vi "AutoDrive.vi"(7 "Drive Params":T1, 8 "Drive PID":T2={"X Dist"={"PID gains"={"proportional gain (Kc)"=1.0, "integral time (Ti, min)"=0.0, "derivative time (Td, min)"=0.0}, "output range"={"output high"=1.0, "output low"=-1.0}}, "Y Dist"={"PID gains"={"proportional gain (Kc)"=1.0, "integral time (Ti, min)"=0.0, "derivative time (Td, min)"=0.0}, "output range"={"output high"=1.0, "output low"=-1.0}}} {"Y Dist"."output range"."output low" format="%.2f"; "Y Dist"."output range"."output high" format="%.2f"; "Y Dist"."PID gains"."derivative time (Td, min)" format="%.3f"; "Y Dist"."PID gains"."integral time (Ti, min)" format="%.3f"; "Y Dist"."PID gains"."proportional gain (Kc)" format="%.3f"; "X Dist"."output range"."output low" format="%.2f"; "X Dist"."output range"."output high" format="%.2f"; "X Dist"."PID gains"."derivative time (Td, min)" format="%.3f"; "X Dist"."PID gains"."integral time (Ti, min)" format="%.3f"; "X Dist"."PID gains"."proportional gain (Kc)" format="%.3f"}, 11 "Array":dbl[](array[numeric]) format="%0.3f") -> (4 "isFinished":bool)   [LabVIEW 2013]
uses:
  AutoDriveParams.ctl
  Drivetrain/DT Mode.ctl
  Drivetrain/Drivetrain Control.ctl
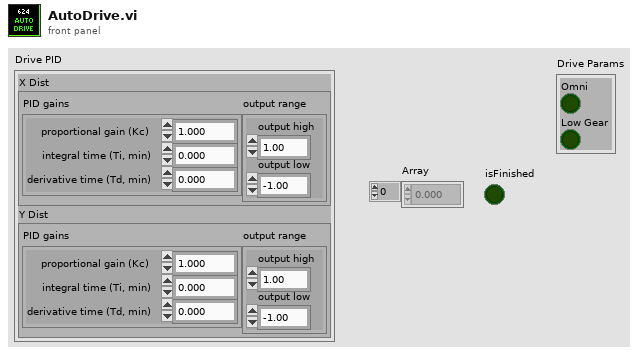
[diagram p1: front panel]
types:
  T1 = typedef "AutoDriveParams.ctl" = cluster{"Omni":bool, "Low Gear":bool}
  T2 = cluster{"X Dist":cluster{"PID gains":cluster{"proportional gain (Kc)":dbl, "integral time (Ti, min)":dbl, "derivative time (Td, min)":dbl}, "output range":cluster{"output high":dbl, "output low":dbl}}, "Y Dist":cluster{"PID gains":cluster{"proportional gain (Kc)":dbl, "integral time (Ti, min)":dbl, "derivative time (Td, min)":dbl}, "output range":cluster{"output high":dbl, "output low":dbl}}}
  T3 = typedef "Drivetrain Control.ctl" = cluster{"axis 1 (x)":dbl, "axis 2 (y)":dbl, "Mode":T4, "heading target":dbl, "steer axis":dbl, "omni?":bool, "Low Gear?":bool, "distance target":cluster{"x":dbl, "y":dbl}, "PID Params":cluster{"X Dist":cluster{"PID gains":cluster{"proportional gain (Kc)":dbl, "integral time (Ti, min)":dbl, "derivative time (Td, min)":dbl}, "output range":cluster{"output high":dbl, "output low":dbl}}, "Y Dist":cluster{"PID gains":cluster{"proportional gain (Kc)":dbl, "integral time (Ti, min)":dbl, "derivative time (Td, min)":dbl}, "output range":cluster{"output high":dbl, "output low":dbl}}}, "Coast":bool}
  T4 = typedef "DT Mode.ctl" = enum16{"Manual", "Gyro Steer", "Distance Drive", "Fieldcentric", "Roll Maneuver", "Alt Roll Maneuver"}
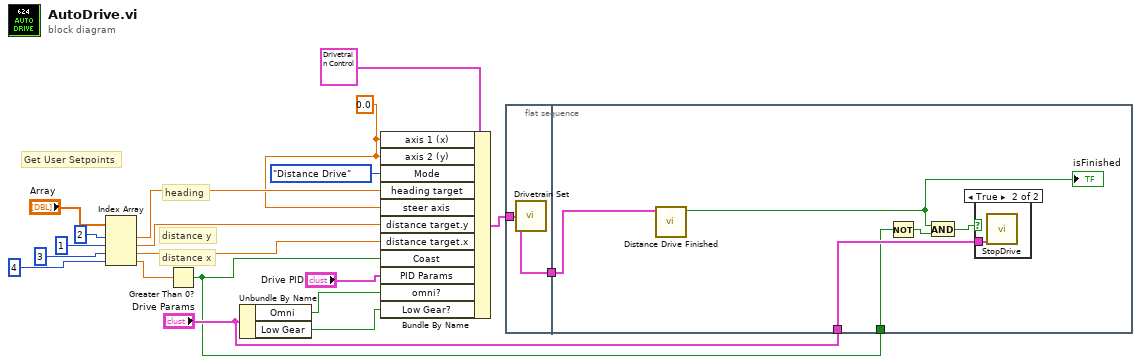
[diagram p0: block diagram]
diagram:
  w8 = 0.0 ("X")
  # "distance x"
  # "distance y"
  # "heading"
  # "Get User Setpoints"
  n1 = Index Array(array="Array", index #1=2 ("index"), index #2=1 ("index"), index #3=3 ("index"), index #4=4 ("index")) -> (element #1=w9:dbl, element #2=w13:dbl, element #3=w11:dbl, element #4=w3:dbl)
  n2 = Greater Than 0?(x=w3) -> (x > 0?=w2:bool)
  n3 = Unbundle By Name("Drive Params") -> ("Omni"=w7:bool, "Low Gear"=w6:bool)
  n4 = Bundle By Name(cluster=T3 {"axis 1 (x)"=0.0, "axis 2 (y)"=0.0, "Mode"=enum."Manual", "heading target"=0.0, "steer axis"=0.0, "omni?"=FALSE, "Low Gear?"=FALSE, "distance target"={"x"=0.0, "y"=0.0}, "PID Params"={"X Dist"={"PID gains"={"proportional gain (Kc)"=0.0, "integral time (Ti, min)"=0.0, "derivative time (Td, min)"=0.0}, "output range"={"output high"=0.0, "output low"=0.0}}, "Y Dist"={"PID gains"={"proportional gain (Kc)"=0.0, "integral time (Ti, min)"=0.0, "derivative time (Td, min)"=0.0}, "output range"={"output high"=0.0, "output low"=0.0}}}, "Coast"=FALSE} ("Drivetrain Control"), "axis 1 (x)"=w8, "axis 2 (y)"=w8, "Mode"=DT_Mode."Distance Drive", "heading target"=w9, "steer axis"=w8, "distance target.y"=w13, "distance target.x"=w11, "Coast"=w2, "PID Params"="Drive PID", "omni?"=w7, "Low Gear?"=w6) -> (w10:T3)
  n5 = flat-sequence {
    tunnel: w10 -> [w20]
    tunnel: [w20] -> w1
    tunnel: "Drive Params" -> [w26]
    tunnel: w2 -> [w23]
    tunnel: w1 -> [w22]
    frame #0 {
      n6 = call "Drivetrain Set.vi"("Drivetrain Control"=w20) -> ()  [unwired: 1 in]
    }
    frame #1 {
      n7 = call "Distance Drive Finished.vi"("Drivetrain Control"=w22) -> ("Finished"=w21:bool)  [unwired: 10 in]
      "isFinished" <- w21
      n8 = Not(x=w23) -> (.not. x?=w24:bool)
      n9 = And(x=w21, y=w24) -> (x .and. y?=w25:bool)
      n10 = case shown="True" w25 {
        tunnel: w26 -> [_ w27]
        frame False {
        }
        frame True {
          n11 = call "StopDrive.vi"("Drive Params"=w27) -> ()  [unwired: 11 in]
        }
      }
    }
  }
